vi "参数设置页.vi"() -> ()   [LabVIEW 2016, in "斯坦道总磷总氮.lvlib"]
uses:
  <vilib>/Plasmionique/MB Master/MB_Master/MB_Master.lvclass
  <vilib>/ptbypt/NI_PtbyPt.lvlib
  <vilib>/Plasmionique/MB Master/MB Master.lvlib
panel:
  in  "手动模式":bool caption="手动模式(hd)"
  in  "简易流程周期设置":cluster{"switch button":bool, "设置按钮":bool}
  out "连接状态":bool
  in  "标样核查自动补测":bool caption="通讯连接"
  in  "跨度核查自动补测":bool caption="通讯连接"
  in  "零点核查自动补测":bool caption="通讯连接"
  in  "标样核查标液偏差":dbl caption="标样核查标液偏差："
  in  "跨度核查标液偏差":dbl caption="跨度核查标液偏差："
  in  "零点核查标液偏差":dbl caption="零点核查标液偏差："
  out "低量程上限":dbl caption="低量程上限：" format="%#_g mg/L"
  in  "简易流程路径":path=path "data/流程.xml"
  out "数据刷新时间":string
  in  "通讯连接":bool=TRUE
  out "MB table":enum32{"Serial", "TCP"}(tab)
  in  "请选择串口:":refnum<visa-resource-name>
  in  "协议":u16(ring)=1 caption="协         议:" items=["斯坦道协议"=1, "国标协议"=2]
  in  "波   特   率:":u32(ring)=115200 items=["115200"=115200, "9600"=9600]
  in  "IP":string="127.0.0.1"
  in  "PORT":string="1001"
  in  "通信方式选择":enum16{"串口", "TCP"}(ring)
  in  "盐度自动补偿：":bool
  out "盐度补偿值":dbl caption="盐度补偿值：" format="%#_g ppt"
  in  "刷新":bool
  in  "测量模式":T1(ring)
  in  "参数下拉列表":u16(ring)
  in  "量程下拉列表":enum16{"低量程", "高量程"}(ring)
  in  "测试流程路径":path=path "data/流程.xml"
  in  "标样核查量程模式":T2 caption="标样核查："
  in  "加标回收量程模式":T2 caption="加标回收："
  in  "跨度核查量程模式":T2 caption="跨度核查："
  in  "零点核查量程模式":T2 caption="零点核查："
  in  "水样测试量程模式":T2 caption="水样测试："
  out "稀释度":dbl caption="稀释度："
  out "阈值（高->低）":dbl caption="阈值（高->低）：" format="%#_g mg/L"
  out "阈值（低->高）":dbl caption="阈值（低->高）：" format="%#_g mg/L"
  out "量程下限":dbl caption="量程下限：" format="%#_g mg/L"
  out "高量程上限":dbl caption="高量程上限：" format="%#_g mg/L"
  out "检出限":dbl caption="检出限：" format="%#_g mg/L"
  out "曲线截距":dbl caption="曲线截距：" format="%#.6f"
  out "曲线斜率":dbl caption="曲线斜率：" format="%#.6f"
  out "二次多项式系数":dbl caption="二次多项式系数：" format="%#.6f"
  out "消解时长":dbl caption="消解时长：" format="%#_g min"
  out "消解温度":dbl caption="消解温度：" format="%#_g ℃"
  out "测量精度":u16 caption="测量精度："
  in  "标样核查标液浓度":dbl caption="标样核查标液浓度："
  in  "跨度核查标液浓度":dbl caption="跨度核查标液浓度："
  in  "零点核查标液浓度":dbl caption="零点核查标液浓度："
  in  "跨度值":dbl caption="跨度值："
  # "日质控设置"
  # "关键参数"
  # "连接设置"
  # "mg/L"
  # "mg/L"
  # "mg/L"
  # "mg/L"
  # "±"
  # "%"
  # "%"
  # "流程设置"
  # "简易流程周期设置"
  # "自动测试量程设置"
  # "设置："
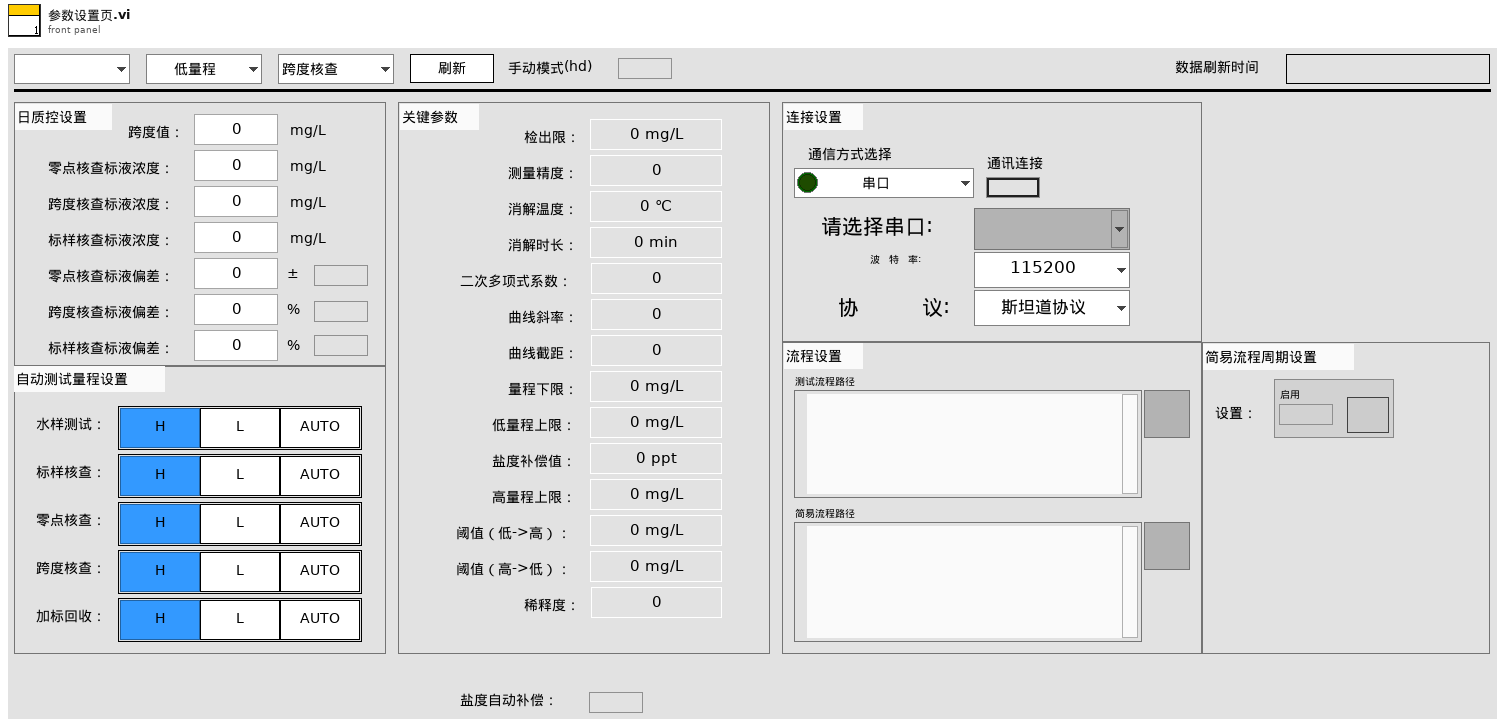
[diagram p1: front panel]
types:
  T1 = enum16{"跨度核查", "水样测量", "零点核查", "标样核查", "加标回收", "平行样测试", "空白校准", "标样校准", "空白测试"}
  T2 = typedef "斯坦道总磷总氮.lvlib/量程模式.ctl" = enum32{"H", "L", "AUTO"}
  T3 = typedef "Cleaning cycle.lvclass/周期项.ctl" = cluster{"时":i32, "分":i32, "频次":string, "id":i32, "参数":string, "simpleflowid":i32, "简易流程名称":string}
  T4 = cluster{"系统时间":timestamp, "工作状态":u16, "测量模式":enum16{"待机", "连续模式", "周期模式", "定点模式", "受控模式", "手动模式"}, "告警代码":u16, "故障代码":u16, "日志代码":u16, "软件版本":u16, "F0":sgl, "F1":sgl, "F2":sgl, "F3":sgl, "T":sgl, "H":sgl, "id":u16, "flowid":u16, "量程":u16, "总磷控温温度1":sgl, "营养盐控温温度2":sgl, "ADC":sgl, "结果值":sgl, "运行时间":u16, "步骤详情":string, "步骤流程":string}
  T5 = typedef "LVStringsAndValuesArrayTypeDef_U16.ctl" = cluster{"String":string, "Value":u16}[]
  T6 = enum8{"Enabled", "Disabled", "Disabled and Grayed Out"}
  T7 = cluster{"测量精度":u16, "检出限":dbl, "上限":dbl, "下限":dbl, "阈值（低->高）":dbl, "阈值（高->低）":dbl, "稀释度":dbl}
  T8 = typedef "操作日志字段定义.ctl" = cluster{"时间":timestamp, "参数":string, "日志信息":string, "流程参数":string}
  T9 = typedef "SingleStepTestV3.lvlib/SingleStepTestV3.lvclass/仪器版本.ctl" = enum16{"V3.1版", "V4版", "V3版", "V4.2版"}
  T10 = typedef "斯坦道总磷总氮.lvlib/V3.1版外设参数.ctl" = cluster{"泵类型":u8, "进样速度":u32, "出样速度":u32, "泵阀量":u8, "阀方向":u8, "光谱仪类型":u8, "光谱采样次数":u8, "氙灯次数":u8, "B":u16, "C":u16, "D":u16, "E":u16, "B_COD":u16, "C_COD":u16, "D_COD":u16, "E_COD":u16, "G":u16, "M":u16, "N":u16, "氨氮注射泵控温下限":sgl, "氨氮注射泵控温上限":sgl, "总氮注射泵控温下限":sgl, "总氮注射泵控温上限":sgl, "消解温度下限":sgl, "消解温度上限":sgl, "加热10s限值":sgl, "KP":sgl, "KI":sgl, "KD":sgl, "高温高压阀开阀温度":sgl, "总氮x公式0":u8, "总氮x公式1":sgl, "总氮x公式2":sgl, "总磷浊度稀释系数":sgl, "总磷浊度补偿权重1":sgl, "总磷浊度补偿权重2":sgl, "盐度系数":sgl, "氨氮补偿系数1":sgl, "氨氮补偿系数2":sgl}
  T11 = typedef "斯坦道总磷总氮.lvlib/V4版外设参数.ctl" = cluster{"泵类型":u8, "注射泵正常速度":u32, "注射泵慢速":u32, "阀型号":u8, "res":u8, "光谱仪类型":u8, "光谱采样次数":u8, "氙灯次数":u8, "B":u16, "C":u16, "D":u16, "E":u16, "B_COD":u16, "C_COD":u16, "D_COD":u16, "E_COD":u16, "G":u16, "M":u16, "N":u16, "降温下限":sgl, "降温上限":sgl, "恒温温度下限":sgl, "恒温温度上限":sgl, "消解温度下限":sgl, "消解温度上限":sgl, "加热10s限值":sgl, "KP":sgl, "KI":sgl, "KD":sgl, "高温高压阀开阀温度":sgl, "总氮x公式0":u8, "总氮x公式1":sgl, "总氮x公式2":sgl, "总磷浊度稀释系数":sgl, "总磷浊度补偿权重1":sgl, "总磷浊度补偿权重2":sgl, "盐度系数":sgl, "氨氮补偿系数1":sgl, "氨氮补偿系数2":sgl, "缺试剂传感器阈值":u16}
  T12 = typedef "斯坦道总磷总氮.lvlib/V4.2版外设参数.ctl" = cluster{"工作模式":u16, "泵类型":u16, "阀型号":u16, "注射泵进样速度":u16, "注射泵出样速度":u16, "注射泵滴定速度":u16, "res":u16, "注射泵慢速":u16, "光谱仪类型":u16, "光谱采样次数":u16, "氙灯次数":u16, "B":u16, "C":u16, "D":u16, "E":u16, "B_COD":u16, "C_COD":u16, "D_COD":u16, "E_COD":u16, "G":u16, "M":u16, "N":u16, "温度校准参数":sgl, "降温温度":sgl, "恒温温度":sgl, "消解温度":sgl, "高温高压阀开阀温度":sgl, "加热超时时间":sgl, "KP":sgl, "KI":sgl, "KD":sgl, "消解PID积分上限":sgl, "恒温PID积分上限":sgl, "PID积分下限":sgl, "缺试剂传感器阈值":u16, "滴定延时":u16, "滴定斜率阈值":sgl, "总氮x公式0":u16, "总氮x公式1":sgl, "总氮x公式2":sgl, "总磷浊度稀释系数":sgl, "总磷浊度补偿权重1":sgl, "总磷浊度补偿权重2":sgl, "盐度系数":sgl, "氨氮补偿系数1":sgl, "氨氮补偿系数2":sgl}
  T13 = typedef "斯坦道总磷总氮.lvlib/V3版外设参数.ctl" = cluster{"泵类型":u8, "进样速度":u32, "出样速度":u32, "泵阀量":u8, "光谱仪类型":u8, "光谱采样次数":u8, "氙灯次数":u8, "B":u16, "C":u16, "D":u16, "E":u16, "B_COD":u16, "C_COD":u16, "D_COD":u16, "E_COD":u16, "G":u16, "M":u16, "N":u16, "氨氮注射泵控温下限":sgl, "氨氮注射泵控温上限":sgl, "总氮注射泵控温下限":sgl, "总氮注射泵控温上限":sgl, "消解温度下限":sgl, "消解温度上限":sgl, "加热10s限值":sgl, "高温高压阀开阀温度":sgl, "总氮x公式0":u8, "总氮x公式1":sgl, "总氮x公式2":sgl, "总磷浊度稀释系数":sgl, "总磷浊度补偿权重1":sgl, "总磷浊度补偿权重2":sgl, "盐度系数":sgl, "氨氮补偿系数1":sgl, "氨氮补偿系数2":sgl}
  T14 = cluster{"水样测试量程模式":T2, "零点核查量程模式":T2, "跨度核查量程模式":T2, "加标回收量程模式":T2, "标样核查量程模式":T2}
  T15 = cluster{"总磷":dbl, "总氮":dbl, "氨氮":dbl, "磷酸盐":dbl, "硝氮":dbl, "亚硝氮":dbl, "硅酸盐":dbl, "硫化物":dbl, "COD":dbl, "氟化物":dbl, "CODMn":dbl}
  T16 = cluster{"总磷跨度值":dbl, "总磷零点标准液浓度":dbl, "总磷跨度标准液浓度":dbl, "总磷标准液标准浓度":dbl, "总氮跨度值":dbl, "总氮零点标准液浓度":dbl, "总氮跨度标准液浓度":dbl, "总氮标准液标准浓度":dbl, "COD跨度值":dbl, "COD零点标准液浓度":dbl, "COD跨度标准液浓度":dbl, "COD标准液标准浓度":dbl, "氨氮跨度值":dbl, "氨氮零点标准液浓度":dbl, "氨氮跨度标准液浓度":dbl, "氨氮标准液标准浓度":dbl, "磷酸盐跨度值":dbl, "磷酸盐零点标准液浓度":dbl, "磷酸盐跨度标准液浓度":dbl, "磷酸盐标准液标准浓度":dbl, "硝氮跨度值":dbl, "硝氮零点标准液浓度":dbl, "硝氮跨度标准液浓度":dbl, "硝氮标准液标准浓度":dbl, "亚硝氮跨度值":dbl, "亚硝氮零点标准液浓度":dbl, "亚硝氮跨度标准液浓度":dbl, "亚硝氮标准液标准浓度":dbl, "硫化物跨度值":dbl, "硫化物零点标准液浓度":dbl, "硫化物跨度标准液浓度":dbl, "硫化物标准液标准浓度":dbl, "硅酸盐跨度值":dbl, "硅酸盐零点标准液浓度":dbl, "硅酸盐跨度标准液浓度":dbl, "硅酸盐标准液标准浓度":dbl, "总磷零点标准液偏差":dbl, "总磷跨度标准液偏差":dbl, "总磷标准液标准偏差":dbl, "总氮零点标准液偏差":dbl, "总氮跨度标准液偏差":dbl, "总氮标准液标准偏差":dbl, "COD零点标准液偏差":dbl, "COD跨度标准液偏差":dbl, "COD标准液标准偏差":dbl, "氨氮零点标准液偏差":dbl, "氨氮跨度标准液偏差":dbl, "氨氮标准液标准偏差":dbl, "磷酸盐零点标准液偏差":dbl, "磷酸盐跨度标准液偏差":dbl, "磷酸盐标准液标准偏差":dbl, "硝氮零点标准液偏差":dbl, "硝氮跨度标准液偏差":dbl, "硝氮标准液标准偏差":dbl, "亚硝氮零点标准液偏差":dbl, "亚硝氮跨度标准液偏差":dbl, "亚硝氮标准液标准偏差":dbl, "硫化物零点标准液偏差":dbl, "硫化物跨度标准液偏差":dbl, "硫化物标准液标准偏差":dbl, "硅酸盐零点标准液偏差":dbl, "硅酸盐跨度标准液偏差":dbl, "硅酸盐标准液标准偏差":dbl, "氟化物跨度值":dbl, "氟化物零点标准液浓度":dbl, "氟化物跨度标准液浓度":dbl, "氟化物标准液标准浓度":dbl, "氟化物零点标准液偏差":dbl, "氟化物跨度标准液偏差":dbl, "氟化物标准液标准偏差":dbl, "CODMn跨度值":dbl, "CODMn零点标准液浓度":dbl, "CODMn跨度标准液浓度":dbl, "CODMn标准液标准浓度":dbl, "CODMn零点标准液偏差":dbl, "CODMn跨度标准液偏差":dbl, "CODMn标准液标准偏差":dbl}
  T17 = cluster{"测量精度":u16, "消解温度":u16, "消解时长":u16, "量程下限":sgl, "量程上限":sgl, "曲线斜率K":sgl, "曲线斜率B":sgl, "标定日期":timestamp, "标液1浓度":sgl, "标液1测量过程值":sgl, "标液2浓度":sgl, "标液2测量过程值":sgl, "标液3浓度":sgl, "标液3测量过程值":sgl, "标液4浓度":sgl, "标液4测量过程值":sgl, "标液5浓度":sgl, "标液5测量过程值":sgl, "线性相关系数":sgl, "试剂余量":u32, "测量滴定值或吸光度":sgl, "空白校准时间":timestamp, "标样校准时间":timestamp, "检出限值":sgl, "校准系数":sgl, "设备系列号":string}
  T18 = cluster{"水样测试量程模式":enum16{"H", "L", "AUTO"}, "空白核查量程模式":enum16{"H", "L", "AUTO"}, "跨度核查量程模式":enum16{"H", "L", "AUTO"}, "加标回收量程模式":enum16{"H", "L", "AUTO"}, "标样核查量程模式":enum16{"H", "L", "AUTO"}}
  T19 = cluster{"水样测试量程模式":u16, "空白核查量程模式":u16, "跨度核查量程模式":u16, "加标回收量程模式":u16, "标样核查量程模式":u16}
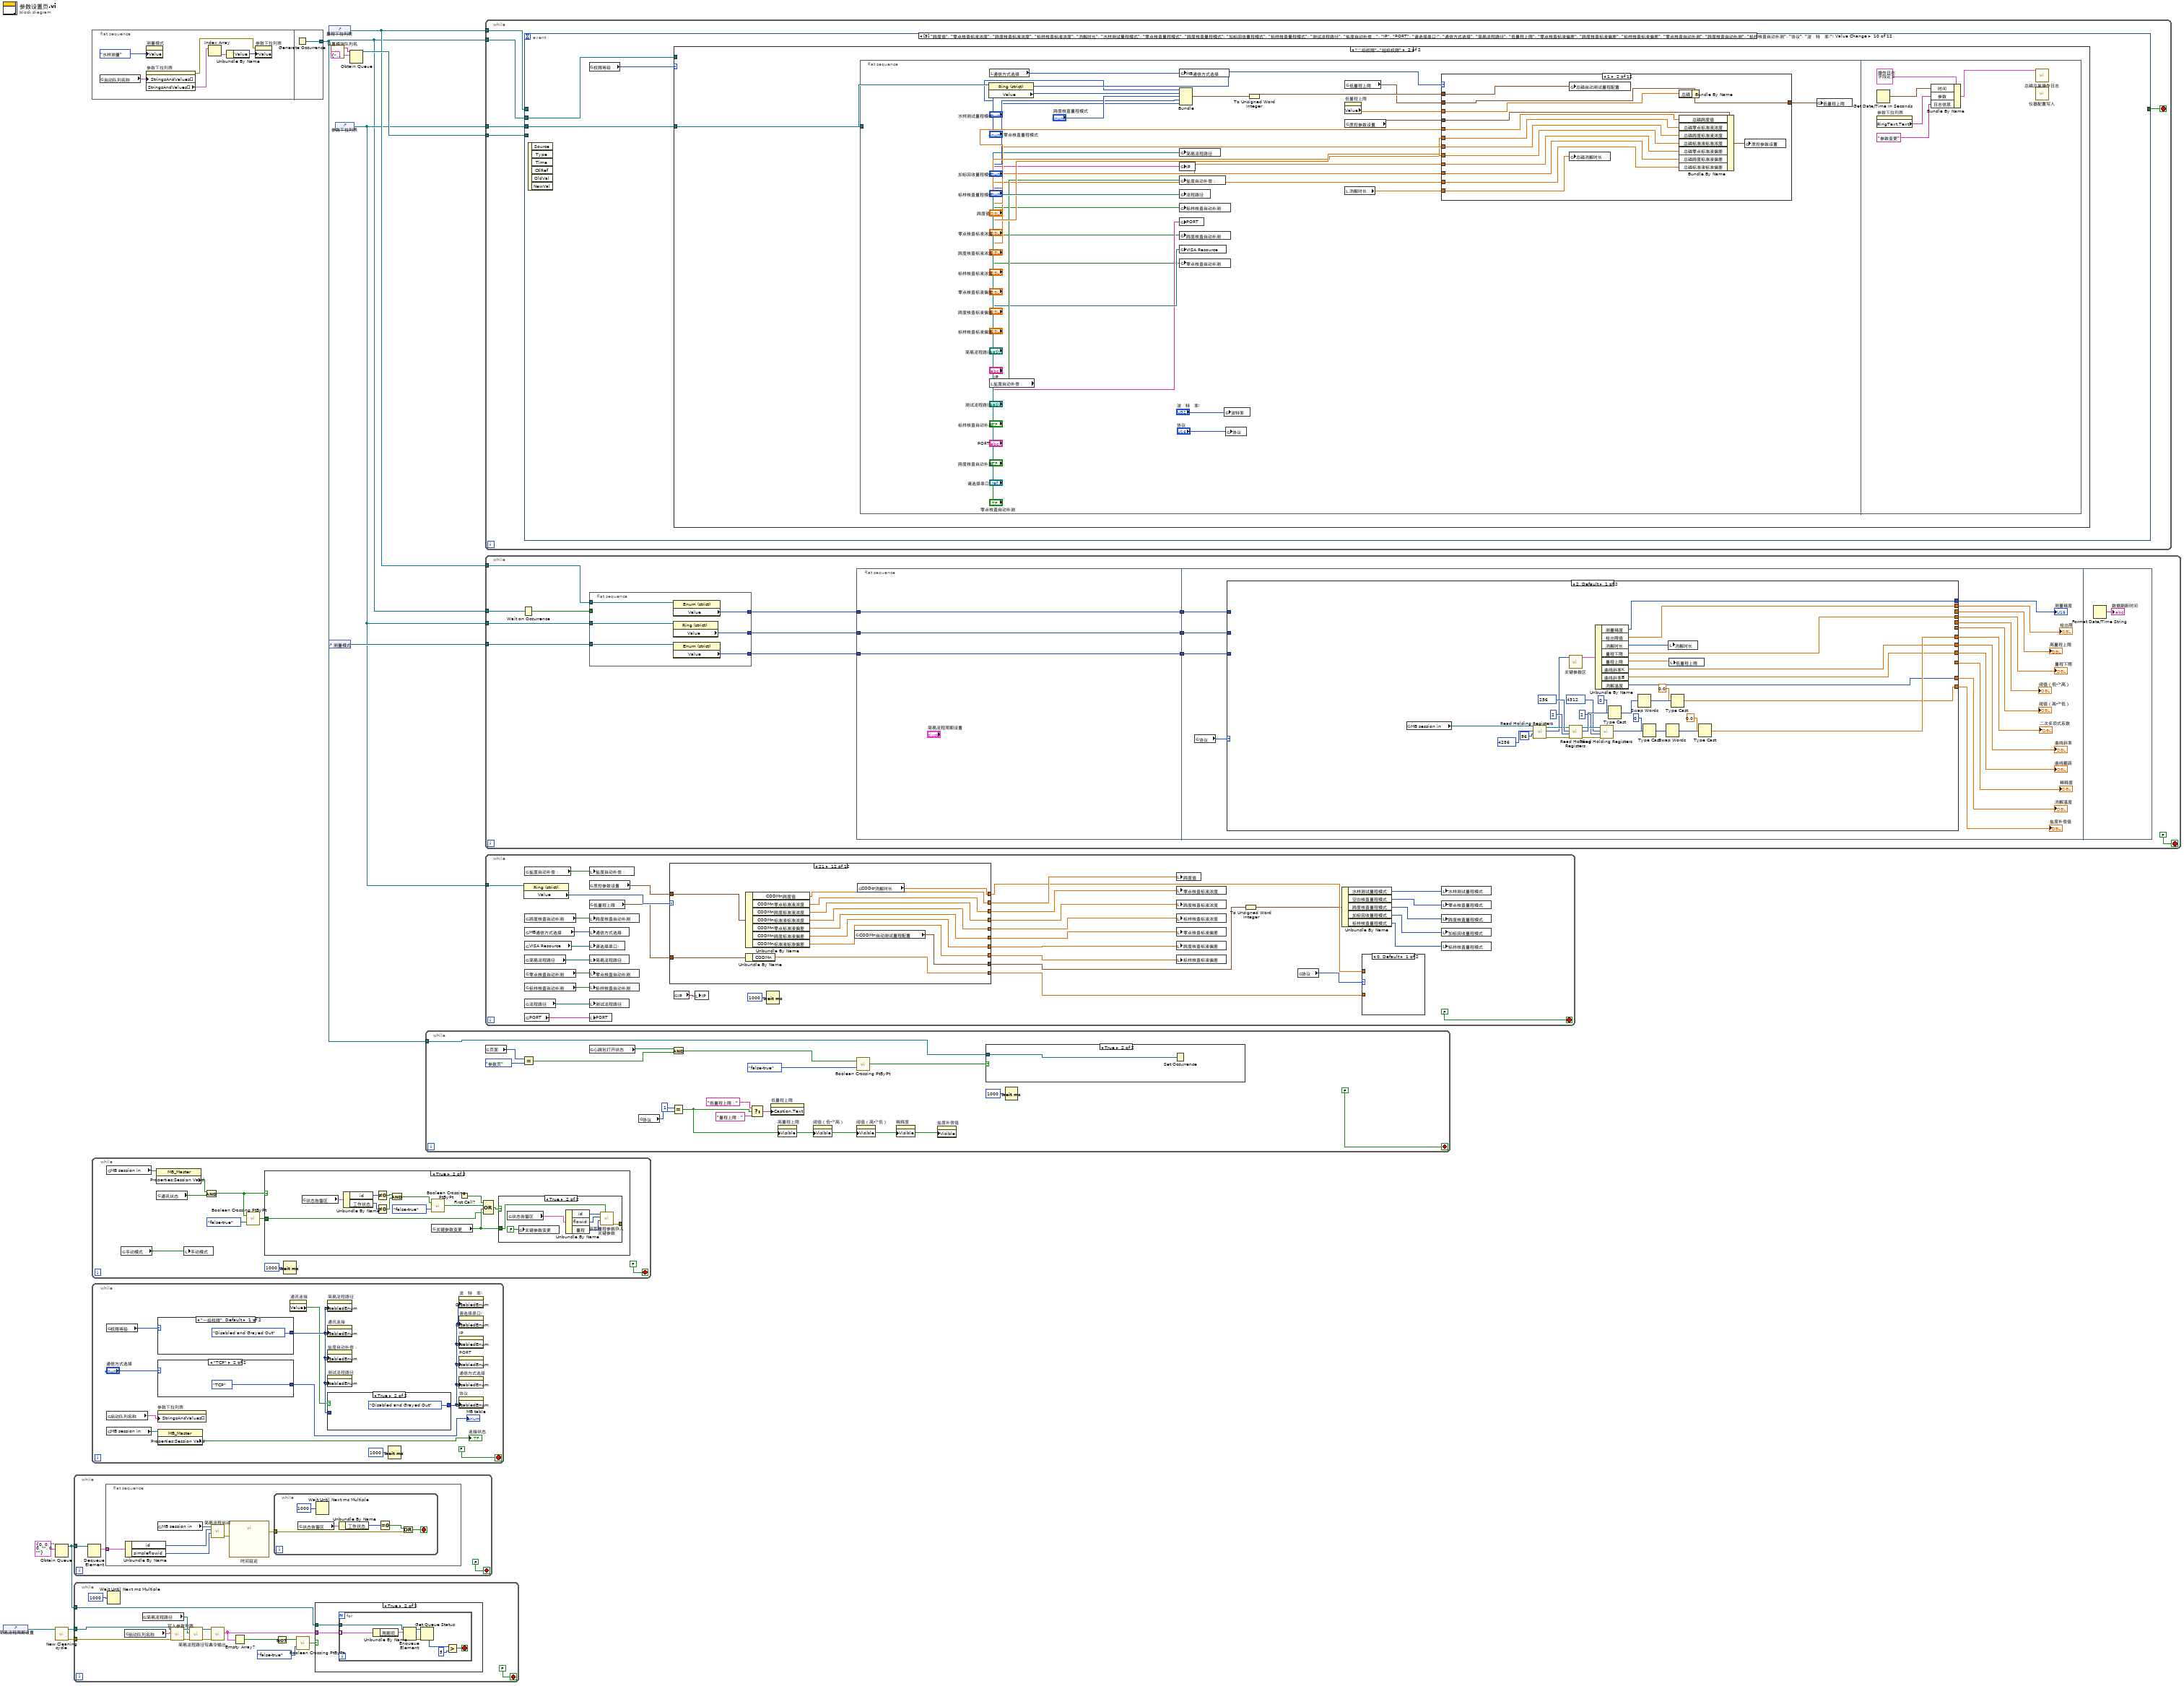
[diagram p0: block diagram]
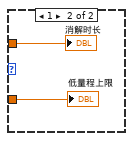
[diagram p6: hidden frame]
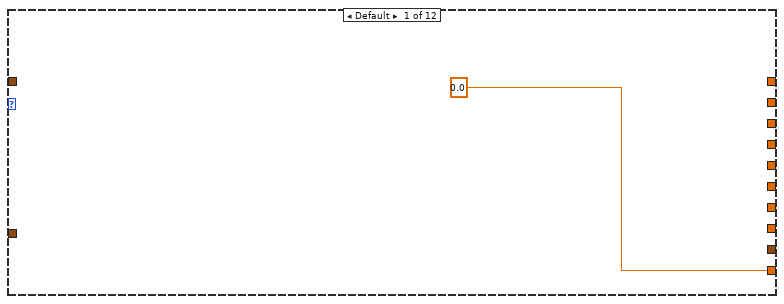
[diagram p7: hidden frame]
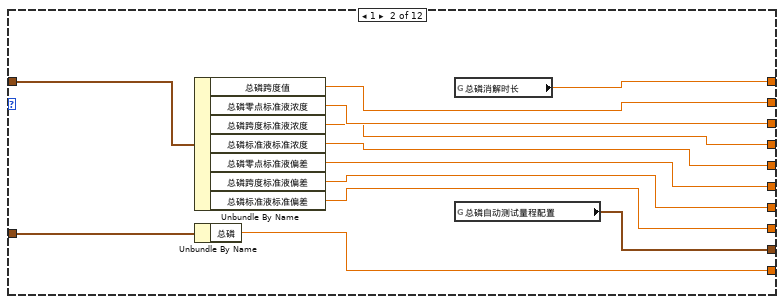
[diagram p8: hidden frame]
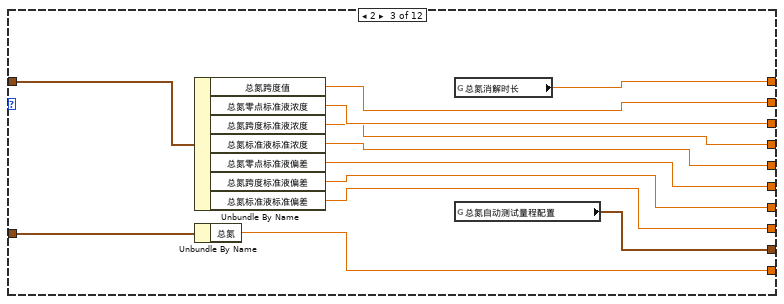
[diagram p9: hidden frame]
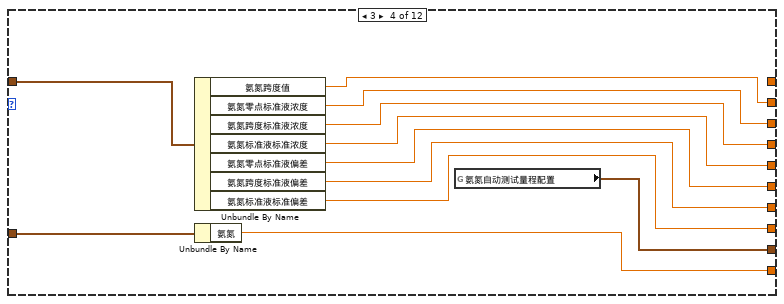
[diagram p10: hidden frame]
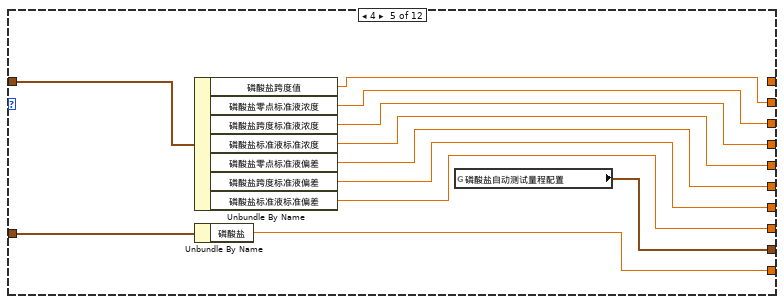
[diagram p11: hidden frame]
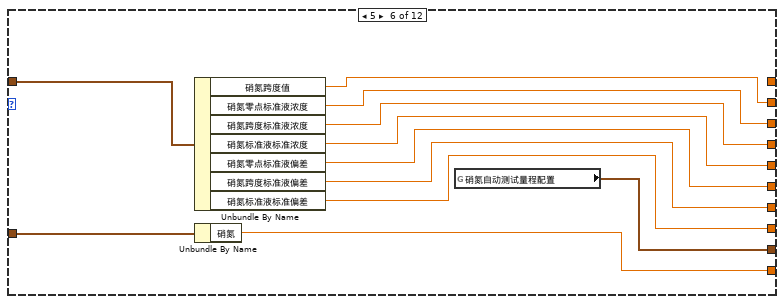
[diagram p12: hidden frame]
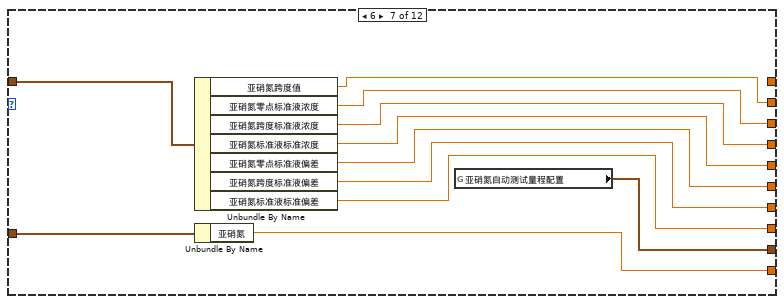
[diagram p13: hidden frame]
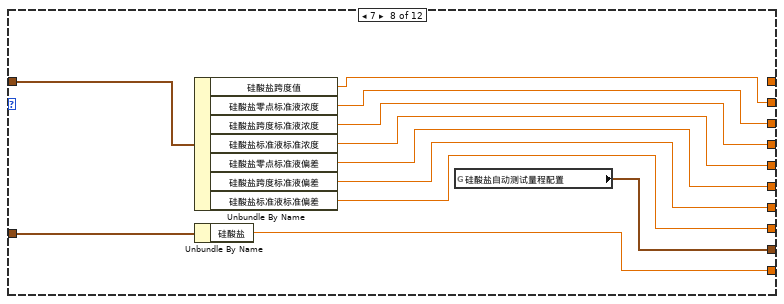
[diagram p14: hidden frame]
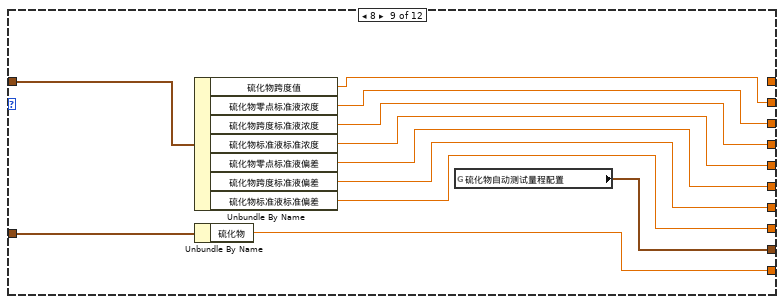
[diagram p15: hidden frame]
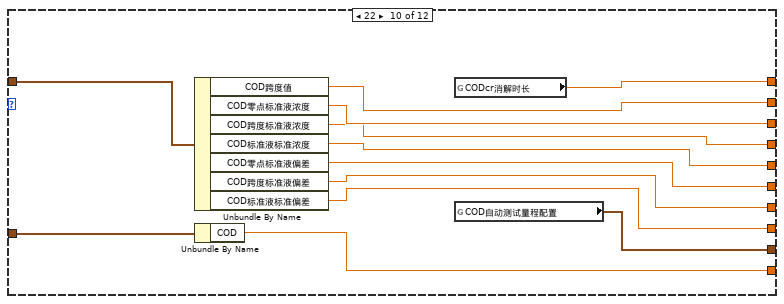
[diagram p16: hidden frame]
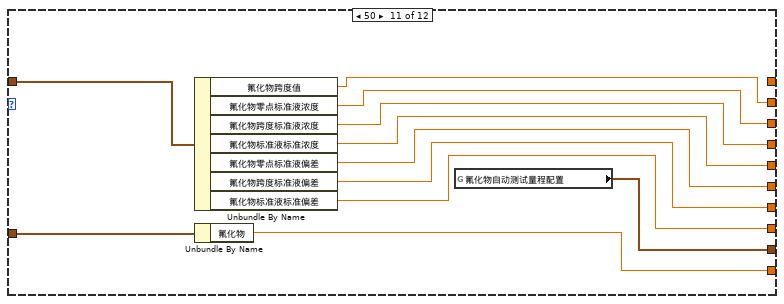
[diagram p17: hidden frame]
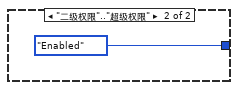
[diagram p18: hidden frame]
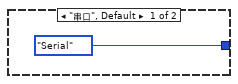
[diagram p19: hidden frame]
diagram:
  n1 = control-ref of="简易流程周期设置"() -> (w3:refnum<vi>)
  n2 = Obtain Queue(element data type=T3 {"时"=0, "分"=0, "频次"="", "id"=0, "参数"="", "simpleflowid"=0, "简易流程名称"=""} ("周期项")) -> (queue out=w1:refnum<queue>)  [unwired: 4 in, 2 out]
  n3 = call "New Cleaning cycle.vi"("Reference"=w3) -> ("error out"=w4:errorcluster, "Cleaningcycle out"=w5:refnum<class "Cleaning cycle.lvclass">)  [unwired: 9 in]
  n4 = while {
    tunnel: w1 -> [w15]
    stop <- FALSE stop-if-true
    n5 = Dequeue Element(queue=w15) -> (element=w14:T3)  [unwired: 2 in, 3 out]
    n6 = flat-sequence {
      tunnel: w14 -> [w20]
      frame #0 {
        n7 = Unbundle By Name(w20) -> ("id"=w18:i32, "simpleflowid"=w19:i32)
        n8 = global read "VAR总磷总氮全局变量.vi" "MB session in"() -> (w21:refnum<class "MB_Master.lvclass">)
        n9 = call "简易流程启动.vi"("简易流程"=w19, "参数Id"=w18, "MB session in"=w21) -> ("error out"=w17:errorcluster)  [unwired: 7 in, 1 out]
        n10 = call "时间延迟"("error in (no error)"=w17) -> ("error out"=w16:errorcluster)  [unwired: 10 in]
        n11 = while {
          tunnel: w16 -> [w23]
          stop <- w22 stop-if-true
          n12 = global read "VAR总磷总氮全局变量.vi" "状态告警区"() -> (w26:T4)
          n13 = Wait Until Next ms Multiple(millisecond multiple=u32 1000 ("毫秒倍数")) -> ()  [unwired: 1 out]
          n14 = Unbundle By Name(w26) -> ("工作状态"=w25:u16)
          n15 = Equal To 0?(x=w25) -> (x = 0?=w24:bool)
          n16 = Or(x=w24, y=w23) -> (x .or. y?=w22:bool)
        }
      }
    }
  }
  n17 = while {
    tunnel: w5 -> [w43]
    tunnel: w4 -> [w42]
    tunnel: w1 -> [w29]
    stop <- FALSE stop-if-true
    n18 = Wait Until Next ms Multiple(millisecond multiple=u32 1000 ("毫秒倍数")) -> ()  [unwired: 1 out]
    n19 = global read "model config var.vi" "启动队列名称"() -> (w39:cluster{"String":string, "Value":u16}[])
    n20 = global read "总磷总氮断电保存全局变量.vi" "简易流程路径"() -> (w38:path)
    n21 = call "写入参数列表.vi"("error in (no error)"=w42, "参数列表"=w39, "Cleaningcycle 输入"=w43) -> ("error out"=w41:errorcluster, "Cleaningcycle 输出"=w40:refnum<class "Cleaning cycle.lvclass">)  [unwired: 7 in]
    n22 = call "简易流程路径写入.vi"("error in (no error)"=w41, "简易流程路径"=w38, "Cleaningcycle 输入"=w40) -> ("error out"=w36:errorcluster, "Cleaningcycle 输出"=w37:refnum<class "Cleaning cycle.lvclass">)  [unwired: 7 in]
    n23 = call "命令输出.vi"("error in (no error)"=w36, "Cleaningcycle 输入"=w37) -> ("命令"=w31:cluster{"触发":bool, "周期项":T3}[])  [unwired: 7 in, 2 out]
    n24 = Empty Array?(array=w31) -> (empty?=w35:bool)
    n25 = Not(x=w35) -> (.not. x?=w34:bool)
    n26 = call <vilib>:"Boolean Crossing PtByPt.vi"("direction"=enum16{"either", "false-true", "true-false"}."false-true", "input"=w34) -> ("crossing"=w32:bool)  [unwired: 1 in]
    n27 = case shown="True" w32 {
      tunnel: w31 -> [_ w45]
      tunnel: w29 -> [_ w44]
      frame False {
      }
      frame True {
        n28 = for {
          tunnel: w45 -> [w53] mode=indexing
          tunnel: w44 -> [w51]
          stop <- w46 stop-if-true
          n29 = Unbundle By Name(w53) -> ("周期项"=w52:T3)
          n30 = Enqueue Element(queue=w51, element=w52) -> (queue out=w50:refnum<queue>, error out=w49:errorcluster)  [unwired: 2 in, 1 out]
          n31 = Get Queue Status(queue=w50, error in (no error)=w49) -> (# elements in queue=w48:i32)  [unwired: 1 in, 7 out]
          n32 = Greater?(x=w48, y=5) -> (0:w46:bool)
        }
      }
    }
  }
  n33 = flat-sequence {
    tunnel: [w60] -> w6
    frame #0 {
      n34 = global read "model config var.vi" "启动队列名称"() -> (w55:cluster{"String":string, "Value":u16}[])
      n35 = property on="测量模式" class="Enum (strict)"("Value"=T1."水样测量" ("测量模式")) -> ()  [unwired: 2 in, 2 out]
      n36 = property on="参数下拉列表" class="Ring (strict)"("StringsAndValues[]"=w55) -> (error out=w58:errorcluster, "StringsAndValues[]"=w56:T5)  [unwired: 2 in, 1 out]
      n37 = Index Array(array=w56) -> (element=w57:cluster{"String":string, "Value":u16})  [unwired: 1 in]
      n38 = Unbundle By Name(w57) -> ("Value"=w59:u16)
      n39 = property on="参数下拉列表" class="Ring (strict)"(error in=w58, "Value"=w59) -> ()  [unwired: 1 in, 2 out]
    }
    frame #1 {
      n40 = Generate Occurrence() -> (w60:refnum<k4>)
    }
  }
  n41 = while {
    stop <- FALSE stop-if-true
    n42 = global read "VAR总磷总氮全局变量.vi" "MB session in"() -> (w66:refnum<class "MB_Master.lvclass">)
    n43 = global read "VAR总磷总氮全局变量.vi" "手动模式"() -> (w61:bool)
    n44 = property class="MB_Master"(reference=w66) -> ("Properties:Session Valid"=w65:bool)  [unwired: 1 in, 2 out]
    n45 = global read "VAR总磷总氮全局变量.vi" "通讯状态"() -> (w68:bool)
    n46 = local write "手动模式"(w61) -> ()
    n47 = And(x=w65, y=w68) -> (x .and. y?=w63:bool)
    n48 = call <vilib>:"Boolean Crossing PtByPt.vi"("direction"=enum16{"either", "false-true", "true-false"}."false-true", "input"=w63) -> ("crossing"=w62:bool)  [unwired: 1 in]
    n49 = case shown="True" w63 {
      tunnel: w62 -> [_ w71]
      frame False {
      }
      frame True {
        n50 = global read "VAR总磷总氮全局变量.vi" "状态告警区"() -> (w81:T4)
        n51 = Unbundle By Name(w81) -> ("id"=w75:u16, "工作状态"=w80:u16)
        n52 = Not Equal To 0?(x=w75) -> (x != 0?=w76:bool)
        n53 = Not Equal To 0?(x=w80) -> (x != 0?=w77:bool)
        n54 = And(x=w76, y=w77) -> (x .and. y?=w78:bool)
        n55 = call <vilib>:"Boolean Crossing PtByPt.vi"("direction"=enum16{"either", "false-true", "true-false"}."false-true", "input"=w78) -> ("crossing"=w74:bool)  [unwired: 1 in]
        n56 = global read "VAR总磷总氮全局变量.vi" "关键参数变更"() -> (w72:bool)
        n57 = First Call?() -> (First Call?: T/F=w70:bool)
        n58 = Compound Arithmetic op=OR ("复合运算")(w70, w74, w72, w71) -> (w73:bool)
        n59 = case shown="True" w73 {
          tunnel: [_ w88] -> _
          tunnel: w72 -> [_ w83]
          frame False {
          }
          frame True {
            n60 = global read "VAR总磷总氮全局变量.vi" "状态告警区"() -> (w87:T4)
            n61 = global write "VAR总磷总氮全局变量.vi" "关键参数变更"(FALSE ("关键参数变更")) -> ()
            n62 = Unbundle By Name(w87) -> ("id"=w86:u16, "flowid"=w85:u16, "量程"=w84:u16)
            n63 = call "获取量程参数存入关键参数.vi"("关键参数变更"=w83, "量程"=w84, "flowid"=w85, "id"=w86) -> ("error out"=w88:errorcluster)  [unwired: 7 in]
          }
        }
      }
    }
    n64 = Wait (ms)(milliseconds to wait=u32 1000 ("等待时间（毫秒）")) -> ()  [unwired: 1 out]
  }
  n65 = while {
    stop <- FALSE stop-if-true
    n66 = global read "VAR总磷总氮全局变量.vi" "权限等级"() -> (w94:enum16{"一级权限", "二级权限", "三级权限", "超级权限"})
    n67 = global read "model config var.vi" "启动队列名称"() -> (w92:cluster{"String":string, "Value":u16}[])
    n68 = global read "VAR总磷总氮全局变量.vi" "MB session in"() -> (w98:refnum<class "MB_Master.lvclass">)
    n69 = case shown="\"一级权限\", Default" w94 {
      tunnel: [T6."Disabled and Grayed Out" ("禁用") T6."Enabled" ("禁用")] -> w93
      frame "一级权限", Default {
      }
      frame "二级权限".."超级权限" {
      }
    }
    n70 = case shown="\"TCP\"" "通信方式选择" {
      tunnel: [enum32{"Serial", "TCP"}."Serial" ("MB table") enum32{"Serial", "TCP"}."TCP" ("MB table")] -> w96
      frame "串口", Default {
      }
      frame "TCP" {
      }
    }
    "MB table" <- w96
    n71 = property on="参数下拉列表" class="Ring (strict)"("StringsAndValues[]"=w92) -> ()  [unwired: 2 in, 2 out]
    n72 = property class="MB_Master"(reference=w98) -> ("Properties:Session Valid"=→"连接状态":bool)  [unwired: 1 in, 2 out]
    n73 = property on="通讯连接" class="Bool (strict)"() -> ("Value"=w90:bool)  [unwired: 2 in, 2 out]
    n74 = property on="简易流程路径" class="Path"("DisabledEnum"=w93) -> ()  [unwired: 2 in, 2 out]
    n75 = property on="通讯连接" class="Bool (strict)"("DisabledEnum"=w93) -> ()  [unwired: 2 in, 2 out]
    n76 = property on="盐度自动补偿：" class="Bool (strict)"("DisabledEnum"=w93) -> ()  [unwired: 2 in, 2 out]
    n77 = property on="测试流程路径" class="Path"("DisabledEnum"=w93) -> ()  [unwired: 2 in, 2 out]
    n78 = case shown="True" w90 {
      tunnel: [w104 T6."Disabled and Grayed Out" ("禁用")] -> w89
      tunnel: w93 -> [w104 _]
      frame False {
      }
      frame True {
      }
    }
    n79 = Wait (ms)(milliseconds to wait=u32 1000 ("等待时间（毫秒）")) -> ()  [unwired: 1 out]
    n80 = property on="波   特   率:" class="Ring (strict)"("DisabledEnum"=w89) -> ()  [unwired: 2 in, 2 out]
    n81 = property on="请选择串口:" class="VISAName"("DisabledEnum"=w89) -> ()  [unwired: 2 in, 2 out]
    n82 = property on="IP" class="Str"("DisabledEnum"=w89) -> ()  [unwired: 2 in, 2 out]
    n83 = property on="PORT" class="Str"("DisabledEnum"=w89) -> ()  [unwired: 2 in, 2 out]
    n84 = property on="通信方式选择" class="Enum (strict)"("DisabledEnum"=w89) -> ()  [unwired: 2 in, 2 out]
    n85 = property on="协议" class="Ring (strict)"("DisabledEnum"=w89) -> ()  [unwired: 2 in, 2 out]
  }
  n86 = control-ref of="量程下拉列表"() -> (w8:refnum<vi>)
  n87 = control-ref of="测量模式"() -> (w9:refnum<vi>)
  n88 = call "设置模块队列名.vi"() -> ("Msg"=w11:string)  [unwired: 5 in]
  n89 = control-ref of="参数下拉列表"() -> (w7:refnum<vi>)
  n90 = Obtain Queue(name (unnamed)=w11, element data type=cluster{"命令":string, "data":variant} {"命令"="", "data"=variant}) -> (queue out=w10:refnum<queue>)  [unwired: 3 in, 2 out]
  n91 = while {
    tunnel: w6 -> [w118]
    stop <- FALSE stop-if-true
    n92 = global read "VAR总磷总氮全局变量.vi" "页面"() -> (w120:enum16{"主页", "参数页", "校准页"})
    n93 = Equal?(x=w120, y=enum16{"主页", "参数页", "校准页"}."参数页" ("页面")) -> (x = y?=w119:bool)
    n94 = global read "VAR总磷总氮全局变量.vi" "心跳包打开状态"() -> (w114:bool)
    n95 = global read "总磷总氮断电保存全局变量.vi" "协议"() -> (w107:u16)
    n96 = And(x=w114, y=w119) -> (x .and. y?=w115:bool)
    n97 = Equal?(x=u16 1, y=w107) -> (x = y?=w108:bool)
    n98 = Select(t="低量程上限：" ("标题.文本"), s=w108, f="量程上限：" ("标题.文本")) -> (s? t:f=w109:string)
    n99 = property on="低量程上限" class="DigNum (strict)"("Caption.Text"=w109) -> ()  [unwired: 2 in, 2 out]
    n100 = property on="高量程上限" class="DigNum (strict)"("Visible"=w108) -> ()  [unwired: 2 in, 2 out]
    n101 = property on="阈值（低->高）" class="DigNum (strict)"("Visible"=w108) -> ()  [unwired: 2 in, 2 out]
    n102 = property on="阈值（高->低）" class="DigNum (strict)"("Visible"=w108) -> ()  [unwired: 2 in, 2 out]
    n103 = call <vilib>:"Boolean Crossing PtByPt.vi"("direction"=enum16{"either", "false-true", "true-false"}."false-true", "input"=w115) -> ("crossing"=w113:bool)  [unwired: 1 in]
    n104 = property on="稀释度" class="DigNum (strict)"("Visible"=w108) -> ()  [unwired: 2 in, 2 out]
    n105 = property on="盐度补偿值" class="DigNum (strict)"("Visible"=w108) -> ()  [unwired: 2 in, 2 out]
    n106 = case shown="True" w113 {
      tunnel: w118 -> [_ w122]
      frame False {
      }
      frame True {
        n107 = Set Occurrence(w122) -> ()
      }
    }
    n108 = Wait (ms)(milliseconds to wait=u32 1000 ("等待时间（毫秒）")) -> ()  [unwired: 1 out]
  }
  n109 = while {
    tunnel: w6 -> [w126]
    tunnel: w7 -> [w125]
    tunnel: w10 -> [w124]
    tunnel: w8 -> [w123]
    stop <- w127 stop-if-true
    n110 = event shown="[9] \"跨度值\", \"零点核查标液浓度\", \"跨度核查标液浓度\", \"标样核查标液浓度\", \"消解时长\", \"水样测试量程模式\", \"零点核查量程模式\", \"跨度核查量程模式\", \"加标回收量程模式\", \"标样核查量程模式\", \"测试流程路径\", \"盐度自动补偿：\", \"IP\", \"PORT\", \"请选择串口:\", \"通信方式选择\", \"简易流程路径\", \"低量程上限\", \"零点核查标液偏差\", \"跨度核查标液偏差\", \"标样核查标液偏差\", \"零点核查自动补测\", \"跨度核查自动补测\", \"标样核查自动补测\", \"协议\", \"波   特   率:\": Value Change" {
      selector: _ -> [_ _ _ _ _ _ _ _ _ _ _ _]
      dyn-events: _ -> [_ _ _ _ _ _ _ _ _ _ _ _]
      timeout: _ -> [_ _ _ _ _ _ _ _ _ _ _ _]
      tunnel: [_ TRUE _ _ _ _ _ _ _ _ _ _] -> w127
      tunnel: w126 -> [_ _ w129 _ _ _ _ _ _ w208 _ _]
      tunnel: w125 -> [_ _ _ _ w148 _ _ _ _ w210 _ _]
      tunnel: w124 -> [_ _ _ _ _ _ _ _ _ _ w400 _]
      tunnel: w123 -> [_ _ _ _ _ _ _ _ _ _ _ _]
      event Timeout {
        n111 = event-data() -> ()  [unwired: 1 in, 3 out]
      }
      event Panel Close {
        n112 = event-data() -> ()  [unwired: 1 in, 4 out]
      }
      event "参数下拉列表", "量程下拉列表", "测量模式", "刷新": Value Change {
        n113 = event-data() -> ()  [unwired: 1 in, 6 out]
        n114 = Set Occurrence(w129) -> ()
      }
      event "跨度值", "零点核查标液浓度", "跨度核查标液浓度", "标样核查标液浓度", "消解温度", "消解时长", "检出限", "高量程上限", "量程下限", "阈值（低->高）", "阈值（高->低）", "稀释度", "低量程上限", "零点核查标液偏差", "跨度核查标液偏差", "标样核查标液偏差": Mouse Down {
        n115 = event-data() -> ("CtlRef"=w131:refnum<vi>)  [unwired: 1 in, 5 out]
        n116 = global read "VAR总磷总氮全局变量.vi" "权限等级"() -> (w130:enum16{"一级权限", "二级权限", "三级权限", "超级权限"})
        n117 = case shown="\"二级权限\"..\"超级权限\"" w130 {
          tunnel: w131 -> [_ w135]
          frame "一级权限", Default {
          }
          frame "二级权限".."超级权限" {
            n118 = property class="DigNum (strict)"(reference=w135) -> (reference out=w133:refnum<vi>, "Value"=w134:dbl)  [unwired: 1 in, 1 out]
            n119 = call "数字键盘.vi"("OldNumber"=w134) -> ("NewNumber"=w132:dbl)
            n120 = property class="DigNum (strict)"(reference=w133, "Val(Sgnl)"=w132) -> ()  [unwired: 1 in, 2 out]
          }
        }
      }
      event "测量精度", "检出限", "高量程上限", "量程下限", "阈值（低->高）", "阈值（高->低）", "稀释度": Value Change {
        n121 = event-data() -> ()  [unwired: 1 in, 6 out]
        n122 = local read "测量精度"() -> (w138:u16)
        n123 = local read "检出限"() -> (w142:dbl)
        n124 = local read "高量程上限"() -> (w144:dbl)
        n125 = local read "量程下限"() -> (w143:dbl)
        n126 = local read "阈值（低->高）"() -> (w141:dbl)
        n127 = local read "阈值（高->低）"() -> (w140:dbl)
        n128 = local read "稀释度"() -> (w139:dbl)
        n129 = property class="Ring (strict)"(reference=w148) -> ("Value"=w147:u16)  [unwired: 1 in, 2 out]
        n130 = Bundle By Name(cluster=T7 {"测量精度"=0, "检出限"=0.0, "上限"=0.0, "下限"=0.0, "阈值（低->高）"=0.0, "阈值（高->低）"=0.0, "稀释度"=0.0} ("量程参数写入"), "测量精度"=w138, "检出限"=w142, "上限"=w144, "下限"=w143, "阈值（低->高）"=w141, "阈值（高->低）"=w140, "稀释度"=w139) -> (w145:T7)
        n131 = call "量程参数写入.vi"("量程参数写入"=w145, "测量参数"=w147) -> ("error out"=w136:errorcluster)  [unwired: 8 in]
        n132 = case shown="No Error" w136 {
          tunnel: ["写入成功" "写入失败"] -> w137
          frame No Error {
            n133 = Get Date/Time In Seconds() -> (seconds since 1Jan1904=w151:timestamp)
            n134 = property on="参数下拉列表" class="Ring (strict)"() -> ("RingText.Text"=w149:string)  [unwired: 2 in, 2 out]
            n135 = Bundle By Name(cluster=T8 {"时间"=timestamp(0 s since 1904-01-01), "参数"="", "日志信息"="", "流程参数"=""} ("data in"), "时间"=w151, "参数"=w149, "日志信息"="关键参数变更") -> (w152:T8)
            n136 = call "总磷总氮操作日志.vi"("data in"=w152) -> ()  [unwired: 10 in, 1 out]
            n137 = global write "VAR总磷总氮全局变量.vi" "关键参数变更"(TRUE ("关键参数变更")) -> ()
          }
          frame Error {
          }
        }
        n138 = One Button Dialog(message=w137) -> ()  [unwired: 1 in, 1 out]
      }
      event "消解温度": Value Change {
        n139 = event-data() -> ("NewVal"=w158:dbl)  [unwired: 1 in, 5 out]
        n140 = global read "VAR总磷总氮全局变量.vi" "MB session in"() -> (w159:refnum<class "MB_Master.lvclass">)
        n141 = call "版本判断.vi"() -> ("仪器版本"=w160:T9)  [unwired: 11 in]
        n142 = case shown="\"V4.2版\"" w160 {
          tunnel: w159 -> [w168 w175 w182 w189]
          tunnel: w158 -> [w163 w171 w178 w185]
          tunnel: [w162 w169 w176 w183] -> w157
          frame "V3.1版", Default {
            n143 = call "读取V3.1外设配置.vi"("MB session in"=w168) -> ("error out"=w164:errorcluster, "外设配置"=w167:T10, "MB session out"=w166:refnum<class "MB_Master.lvclass">)  [unwired: 8 in]
            n144 = Bundle By Name(cluster=w167, "消解温度下限"=w163) -> (w165:T10)
            n145 = call "写入V3.1外设配置.vi"("error in (no error)"=w164, "外设配置"=w165, "MB session in"=w166) -> ("error out"=w162:errorcluster)  [unwired: 7 in, 1 out]
          }
          frame "V4版" {
            n146 = call "读取V4版外设配置.vi"("MB session in"=w175) -> ("error out"=w170:errorcluster, "外设配置"=w173:T11, "MB session out"=w174:refnum<class "MB_Master.lvclass">)  [unwired: 8 in]
            n147 = Bundle By Name(cluster=w173, "消解温度下限"=w171) -> (w172:T11)
            n148 = call "写入V4版外设配置.vi"("error in (no error)"=w170, "外设配置"=w172, "MB session in"=w174) -> ("error out"=w169:errorcluster)  [unwired: 7 in, 1 out]
          }
          frame "V4.2版" {
            n149 = call "读取V4.2版外设配置.vi"("MB session in"=w182) -> ("error out"=w177:errorcluster, "外设配置"=w180:T12, "MB session out"=w181:refnum<class "MB_Master.lvclass">)  [unwired: 8 in]
            n150 = Bundle By Name(cluster=w180, "消解温度"=w178) -> (w179:T12)
            n151 = call "写入V4.2版外设配置.vi"("error in (no error)"=w177, "外设配置"=w179, "MB session in"=w181) -> ("error out"=w176:errorcluster)  [unwired: 7 in, 1 out]
          }
          frame "V3版" {
            n152 = call "读取V3外设配置.vi"("MB session in"=w189) -> ("error out"=w184:errorcluster, "外设配置"=w187:T13, "MB session out"=w188:refnum<class "MB_Master.lvclass">)  [unwired: 8 in]
            n153 = Bundle By Name(cluster=w187, "消解温度下限"=w185) -> (w186:T13)
            n154 = call "写入V3外设配置.vi"("error in (no error)"=w184, "外设配置"=w186, "MB session in"=w188) -> ("error out"=w183:errorcluster)  [unwired: 7 in, 1 out]
          }
        }
        n155 = case shown="Error" w157 {
          tunnel: ["写入成功" "写入失败"] -> w161
          frame No Error {
          }
          frame Error {
          }
        }
        n156 = One Button Dialog(message=w161) -> ()  [unwired: 1 in, 1 out]
      }
      event "测量精度": Mouse Down {
        n157 = event-data() -> ("CtlRef"=w193:refnum<vi>)  [unwired: 1 in, 7 out]
        n158 = global read "VAR总磷总氮全局变量.vi" "权限等级"() -> (w192:enum16{"一级权限", "二级权限", "三级权限", "超级权限"})
        n159 = case shown="\"二级权限\"..\"超级权限\"" w192 {
          tunnel: w193 -> [_ w197]
          frame "一级权限", Default {
          }
          frame "二级权限".."超级权限" {
            n160 = property class="DigNum (strict)"(reference=w197) -> (reference out=w195:refnum<vi>, "Value"=w196:u16)  [unwired: 1 in, 1 out]
            n161 = call "数字键盘.vi"("OldNumber"=w196) -> ("NewNumber"=w194:dbl)
            n162 = property class="DigNum (strict)"(reference=w195, "Val(Sgnl)"=w194) -> ()  [unwired: 1 in, 2 out]
          }
        }
      }
      event "盐度补偿值": Mouse Down {
        n163 = event-data() -> ("CtlRef"=w199:refnum<vi>)  [unwired: 1 in, 3 out]
        n164 = global read "VAR总磷总氮全局变量.vi" "权限等级"() -> (w198:enum16{"一级权限", "二级权限", "三级权限", "超级权限"})
        n165 = case shown="\"二级权限\"..\"超级权限\"" w198 {
          tunnel: w199 -> [_ w201]
          frame "一级权限", Default {
          }
          frame "二级权限".."超级权限" {
            n166 = case shown="False" "盐度自动补偿：" {
              tunnel: w201 -> [w205 _]
              frame False {
                n167 = property class="DigNum (strict)"(reference=w205) -> (reference out=w203:refnum<vi>, "Value"=w204:dbl)  [unwired: 1 in, 1 out]
                n168 = call "数字键盘.vi"("OldNumber"=w204) -> ("NewNumber"=w202:dbl)
                n169 = property class="DigNum (strict)"(reference=w203, "Val(Sgnl)"=w202) -> ()  [unwired: 1 in, 2 out]
              }
              frame True {
              }
            }
          }
        }
      }
      event "盐度补偿值": Value Change {
        n170 = event-data() -> ("NewVal"=w206:dbl)  [unwired: 1 in, 5 out]
        n171 = global read "VAR总磷总氮全局变量.vi" "MB session in"() -> (w207:refnum<class "MB_Master.lvclass">)
        n172 = call "盐度补偿值写入.vi"("盐度补偿值"=w206, "MB session in"=w207) -> ()  [unwired: 8 in, 2 out]
      }
      event "跨度值", "零点核查标液浓度", "跨度核查标液浓度", "标样核查标液浓度", "消解时长", "测试流程路径", "盐度自动补偿：", "IP", "PORT", "请选择串口:", "通信方式选择", "简易流程路径", "低量程上限", "零点核查标液偏差", "跨度核查标液偏差", "标样核查标液偏差", "零点核查自动补测", "跨度核查自动补测", "标样核查自动补测", "协议", "波   特   率:": Value Change {
        n173 = event-data() -> ()  [unwired: 1 in, 6 out]
        n174 = global read "VAR总磷总氮全局变量.vi" "权限等级"() -> (w209:enum16{"一级权限", "二级权限", "三级权限", "超级权限"})
        n175 = case shown="\"二级权限\"..\"超级权限\"" w209 {
          tunnel: w210 -> [_ w212]
          tunnel: w208 -> [w211 _]
          frame "一级权限", Default {
            n176 = Set Occurrence(w211) -> ()
          }
          frame "二级权限".."超级权限" {
            n177 = flat-sequence {
              tunnel: w212 -> [w244]
              frame #0 {
                n178 = property class="Ring (strict)"(reference=w244) -> ("Value"=w243:u16)  [unwired: 1 in, 2 out]
                n179 = local read "通信方式选择"() -> (w226:enum16{"串口", "TCP"})
                n180 = local read "盐度自动补偿："() -> (w230:bool)
                n181 = global write "总磷总氮断电保存全局变量.vi" "MB通信方式选择"(w226) -> ()
                n182 = Bundle("水样测试量程模式"="水样测试量程模式", "零点核查量程模式"="零点核查量程模式", "跨度核查量程模式"="跨度核查量程模式", "加标回收量程模式"="加标回收量程模式", "标样核查量程模式"="标样核查量程模式") -> (w232:T14)  [unwired: 1 in]
                n183 = global write "总磷总氮断电保存全局变量.vi" "简易流程路径"("简易流程路径") -> ()
                n184 = global write "总磷总氮断电保存全局变量.vi" "IP"("IP") -> ()
                n185 = global write "总磷总氮断电保存全局变量.vi" "盐度自动补偿："(w230) -> ()
                n186 = global write "总磷总氮断电保存全局变量.vi" "流程路径"("测试流程路径") -> ()
                n187 = global write "总磷总氮断电保存全局变量.vi" "标样核查自动补测"("标样核查自动补测") -> ()
                n188 = global write "总磷总氮断电保存全局变量.vi" "PORT"("PORT") -> ()
                n189 = global write "总磷总氮断电保存全局变量.vi" "跨度核查自动补测"("跨度核查自动补测") -> ()
                n190 = global write "总磷总氮断电保存全局变量.vi" "VISA Resource"("请选择串口:") -> ()
                n191 = global write "总磷总氮断电保存全局变量.vi" "零点核查自动补测"("零点核查自动补测") -> ()
                n192 = global write "总磷总氮断电保存全局变量.vi" "波特率"("波   特   率:") -> ()
                n193 = global write "总磷总氮断电保存全局变量.vi" "协议"("协议") -> ()
                n194 = To Unsigned Word Integer(number=w232) -> (unsigned 16bit integer=w231:cluster{u16, u16, u16, u16, u16})
                n195 = global read "总磷总氮断电保存全局变量.vi" "低量程上限"() -> (w223:T15)
                n196 = property on="低量程上限" class="DigNum (strict)"() -> ("Value"=w221:dbl)  [unwired: 2 in, 2 out]
                n197 = global read "总磷总氮断电保存全局变量.vi" "质控参数设置"() -> (w238:T16)
                n198 = local read "消解时长"() -> (w225:dbl)
                n199 = case shown="1" w243 {
                  tunnel: "跨度值" -> [_ w258 w272 w285 w298 w311 w324 w337 w350 w364 w378 w391]
                  tunnel: "标样核查标液浓度" -> [_ w255 w269 w282 w295 w308 w321 w334 w347 w361 w375 w388]
                  tunnel: "跨度核查标液浓度" -> [_ w256 w270 w283 w296 w309 w322 w335 w348 w362 w376 w389]
                  tunnel: "零点核查标液浓度" -> [_ w257 w271 w284 w297 w310 w323 w336 w349 w363 w377 w390]
                  tunnel: w238 -> [_ w260 w274 w287 w300 w313 w326 w339 w352 w366 w380 w393]
                  tunnel: w231 -> [_ w254 w268 w281 w294 w307 w320 w333 w346 w359 w373 w387]
                  tunnel: w225 -> [_ w253 w267 _ _ _ _ _ _ w360 w374 _]
                  tunnel: w223 -> [w246 w251 w266 w280 w293 w306 w319 w332 w345 w358 w372 w386]
                  tunnel: [w246 w250 w264 w279 w292 w305 w318 w331 w344 w357 w371 w385] -> w222
                  tunnel: w221 -> [_ w252 w265 w278 w291 w304 w317 w330 w343 w356 w370 w384]
                  tunnel: "标样核查标液偏差" -> [_ w249 w261 w275 w288 w303 w314 w327 w340 w353 w367 w381]
                  tunnel: "跨度核查标液偏差" -> [_ w248 w262 w276 w289 w302 w315 w328 w341 w354 w368 w382]
                  tunnel: "零点核查标液偏差" -> [_ w247 w263 w277 w290 w301 w316 w329 w342 w355 w369 w383]
                  frame 0, Default {
                  }
                  frame 1 {
                    n200 = global write "总磷总氮断电保存全局变量.vi" "总磷自动测试量程配置"(w254) -> ()
                    n201 = global write "总磷总氮断电保存全局变量.vi" "总磷消解时长"(w253) -> ()
                    n202 = Bundle By Name(cluster=w251, "总磷"=w252) -> (w250:T15)
                    n203 = Bundle By Name(cluster=w260, "总磷跨度值"=w258, "总磷零点标准液浓度"=w257, "总磷跨度标准液浓度"=w256, "总磷标准液标准浓度"=w255, "总磷零点标准液偏差"=w247, "总磷跨度标准液偏差"=w248, "总磷标准液标准偏差"=w249) -> (w259:T16)
                    n204 = global write "总磷总氮断电保存全局变量.vi" "质控参数设置"(w259) -> ()
                  }
                  frame 2 {
                    n205 = global write "总磷总氮断电保存全局变量.vi" "总氮自动测试量程配置"(w268) -> ()
                    n206 = global write "总磷总氮断电保存全局变量.vi" "总氮消解时长"(w267) -> ()
                    n207 = Bundle By Name(cluster=w266, "总氮"=w265) -> (w264:T15)
                    n208 = Bundle By Name(cluster=w274, "总氮跨度值"=w272, "总氮零点标准液浓度"=w271, "总氮跨度标准液浓度"=w270, "总氮标准液标准浓度"=w269, "总氮零点标准液偏差"=w263, "总氮跨度标准液偏差"=w262, "总氮标准液标准偏差"=w261) -> (w273:T16)
                    n209 = global write "总磷总氮断电保存全局变量.vi" "质控参数设置"(w273) -> ()
                  }
                  frame 3 {
                    n210 = global write "总磷总氮断电保存全局变量.vi" "氨氮自动测试量程配置"(w281) -> ()
                    n211 = Bundle By Name(cluster=w280, "氨氮"=w278) -> (w279:T15)
                    n212 = Bundle By Name(cluster=w287, "氨氮跨度值"=w285, "氨氮零点标准液浓度"=w284, "氨氮跨度标准液浓度"=w283, "氨氮标准液标准浓度"=w282, "氨氮零点标准液偏差"=w277, "氨氮跨度标准液偏差"=w276, "氨氮标准液标准偏差"=w275) -> (w286:T16)
                    n213 = global write "总磷总氮断电保存全局变量.vi" "质控参数设置"(w286) -> ()
                  }
                  frame 4 {
                    n214 = global write "总磷总氮断电保存全局变量.vi" "磷酸盐自动测试量程配置"(w294) -> ()
                    n215 = Bundle By Name(cluster=w293, "磷酸盐"=w291) -> (w292:T15)
                    n216 = Bundle By Name(cluster=w300, "磷酸盐跨度值"=w298, "磷酸盐零点标准液浓度"=w297, "磷酸盐跨度标准液浓度"=w296, "磷酸盐标准液标准浓度"=w295, "磷酸盐零点标准液偏差"=w290, "磷酸盐跨度标准液偏差"=w289, "磷酸盐标准液标准偏差"=w288) -> (w299:T16)
                    n217 = global write "总磷总氮断电保存全局变量.vi" "质控参数设置"(w299) -> ()
                  }
                  frame 5 {
                    n218 = global write "总磷总氮断电保存全局变量.vi" "硝氮自动测试量程配置"(w307) -> ()
                    n219 = Bundle By Name(cluster=w306, "硝氮"=w304) -> (w305:T15)
                    n220 = Bundle By Name(cluster=w313, "硝氮跨度值"=w311, "硝氮零点标准液浓度"=w310, "硝氮跨度标准液浓度"=w309, "硝氮标准液标准浓度"=w308, "硝氮零点标准液偏差"=w301, "硝氮跨度标准液偏差"=w302, "硝氮标准液标准偏差"=w303) -> (w312:T16)
                    n221 = global write "总磷总氮断电保存全局变量.vi" "质控参数设置"(w312) -> ()
                  }
                  frame 6 {
                    n222 = global write "总磷总氮断电保存全局变量.vi" "亚硝氮自动测试量程配置"(w320) -> ()
                    n223 = Bundle By Name(cluster=w319, "亚硝氮"=w317) -> (w318:T15)
                    n224 = Bundle By Name(cluster=w326, "亚硝氮跨度值"=w324, "亚硝氮零点标准液浓度"=w323, "亚硝氮跨度标准液浓度"=w322, "亚硝氮标准液标准浓度"=w321, "亚硝氮零点标准液偏差"=w316, "亚硝氮跨度标准液偏差"=w315, "亚硝氮标准液标准偏差"=w314) -> (w325:T16)
                    n225 = global write "总磷总氮断电保存全局变量.vi" "质控参数设置"(w325) -> ()
                  }
                  frame 7 {
                    n226 = global write "总磷总氮断电保存全局变量.vi" "硅酸盐自动测试量程配置"(w333) -> ()
                    n227 = Bundle By Name(cluster=w332, "硅酸盐"=w330) -> (w331:T15)
                    n228 = Bundle By Name(cluster=w339, "硅酸盐跨度值"=w337, "硅酸盐零点标准液浓度"=w336, "硅酸盐跨度标准液浓度"=w335, "硅酸盐标准液标准浓度"=w334, "硅酸盐零点标准液偏差"=w329, "硅酸盐跨度标准液偏差"=w328, "硅酸盐标准液标准偏差"=w327) -> (w338:T16)
                    n229 = global write "总磷总氮断电保存全局变量.vi" "质控参数设置"(w338) -> ()
                  }
                  frame 8 {
                    n230 = global write "总磷总氮断电保存全局变量.vi" "硫化物自动测试量程配置"(w346) -> ()
                    n231 = Bundle By Name(cluster=w345, "硫化物"=w343) -> (w344:T15)
                    n232 = Bundle By Name(cluster=w352, "硫化物跨度值"=w350, "硫化物零点标准液浓度"=w349, "硫化物跨度标准液浓度"=w348, "硫化物标准液标准浓度"=w347, "硫化物零点标准液偏差"=w342, "硫化物跨度标准液偏差"=w341, "硫化物标准液标准偏差"=w340) -> (w351:T16)
                    n233 = global write "总磷总氮断电保存全局变量.vi" "质控参数设置"(w351) -> ()
                  }
                  frame 22 {
                    n234 = global write "总磷总氮断电保存全局变量.vi" "COD自动测试量程配置"(w359) -> ()
                    n235 = global write "总磷总氮断电保存全局变量.vi" "CODcr消解时长"(w360) -> ()
                    n236 = Bundle By Name(cluster=w358, "COD"=w356) -> (w357:T15)
                    n237 = Bundle By Name(cluster=w366, "COD跨度值"=w364, "COD零点标准液浓度"=w363, "COD跨度标准液浓度"=w362, "COD标准液标准浓度"=w361, "COD零点标准液偏差"=w355, "COD跨度标准液偏差"=w354, "COD标准液标准偏差"=w353) -> (w365:T16)
                    n238 = global write "总磷总氮断电保存全局变量.vi" "质控参数设置"(w365) -> ()
                  }
                  frame 21 {
                    n239 = global write "总磷总氮断电保存全局变量.vi" "CODMn自动测试量程配置"(w373) -> ()
                    n240 = global write "总磷总氮断电保存全局变量.vi" "CODmn消解时长"(w374) -> ()
                    n241 = Bundle By Name(cluster=w372, "CODMn"=w370) -> (w371:T15)
                    n242 = Bundle By Name(cluster=w380, "CODMn跨度值"=w378, "CODMn零点标准液浓度"=w377, "CODMn跨度标准液浓度"=w376, "CODMn标准液标准浓度"=w375, "CODMn零点标准液偏差"=w369, "CODMn跨度标准液偏差"=w368, "CODMn标准液标准偏差"=w367) -> (w379:T16)
                    n243 = global write "总磷总氮断电保存全局变量.vi" "质控参数设置"(w379) -> ()
                  }
                  frame 50 {
                    n244 = global write "总磷总氮断电保存全局变量.vi" "氟化物自动测试量程配置"(w387) -> ()
                    n245 = Bundle By Name(cluster=w386, "氟化物"=w384) -> (w385:T15)
                    n246 = Bundle By Name(cluster=w393, "氟化物跨度值"=w391, "氟化物零点标准液浓度"=w390, "氟化物跨度标准液浓度"=w389, "氟化物标准液标准浓度"=w388, "氟化物零点标准液偏差"=w383, "氟化物跨度标准液偏差"=w382, "氟化物标准液标准偏差"=w381) -> (w392:T16)
                    n247 = global write "总磷总氮断电保存全局变量.vi" "质控参数设置"(w392) -> ()
                  }
                }
                n248 = global write "总磷总氮断电保存全局变量.vi" "低量程上限"(w222) -> ()
              }
              frame #1 {
                n249 = Get Date/Time In Seconds() -> (seconds since 1Jan1904=w396:timestamp)
                n250 = property on="参数下拉列表" class="Ring (strict)"() -> ("RingText.Text"=w394:string)  [unwired: 2 in, 2 out]
                n251 = Bundle By Name(cluster=T8 {"时间"=timestamp(0 s since 1904-01-01), "参数"="", "日志信息"="", "流程参数"=""} ("data in"), "时间"=w396, "参数"=w394, "日志信息"="参数变更") -> (w397:T8)
                n252 = call "总磷总氮操作日志.vi"("data in"=w397) -> ()  [unwired: 10 in, 1 out]
                n253 = call "仪器配置写入.vi"() -> ()  [unwired: 11 in, 1 out]
              }
            }
          }
        }
      }
      event "通讯连接": Value Change {
        n254 = event-data() -> ("NewVal"=w399:bool)  [unwired: 1 in, 5 out]
        n255 = Flush Queue(queue=w400) -> (queue out=w401:refnum<queue>)  [unwired: 1 in, 2 out]
        n256 = case shown="False" w399 {
          tunnel: w401 -> [w402 w404]
          frame False {
            n257 = Enqueue Element At Opposite End(queue=w402, element=cluster{"命令":string, "data":variant} {"命令"="停用模块", "data"=variant} ("元素")) -> ()  [unwired: 2 in, 3 out]
          }
          frame True {
            n258 = Enqueue Element At Opposite End(queue=w404, element=cluster{"命令":string, "data":variant} {"命令"="启用模块", "data"=variant} ("元素")) -> ()  [unwired: 2 in, 3 out]
          }
        }
      }
      event "手动模式": Value Change {
        n259 = event-data() -> ()  [unwired: 1 in, 6 out]
        n260 = global write "VAR总磷总氮全局变量.vi" "手动模式"("手动模式") -> ()
      }
    }
  }
  n261 = while {
    tunnel: w7 -> [w417]
    tunnel: w8 -> [w416]
    tunnel: w9 -> [w415]
    tunnel: w6 -> [w414]
    stop <- FALSE stop-if-true
    n262 = Wait on Occurrence(2:w414) -> (0:w408:bool)  [unwired: 2 in]
    n263 = flat-sequence {
      tunnel: w417 -> [w424]
      tunnel: w416 -> [w423]
      tunnel: w415 -> [w422]
      tunnel: [w421] -> w411
      tunnel: [w420] -> w410
      tunnel: [w419] -> w409
      tunnel: w408 -> [_]
      frame #0 {
        n264 = property class="Enum (strict)"(reference=w423) -> ("Value"=w420:enum16{"低量程", "高量程"})  [unwired: 1 in, 2 out]
        n265 = property class="Ring (strict)"(reference=w424) -> ("Value"=w421:u16)  [unwired: 1 in, 2 out]
        n266 = property class="Enum (strict)"(reference=w422) -> ("Value"=w419:T1)  [unwired: 1 in, 2 out]
      }
    }
    n267 = flat-sequence {
      tunnel: [w427] -> w413
      tunnel: [w426] -> w412
      tunnel: w411 -> [w425]
      tunnel: w410 -> [w427]
      tunnel: w409 -> [w426]
      tunnel: [w425] -> w407
      tunnel: w413 -> [w442]
      tunnel: w412 -> [w443]
      tunnel: w407 -> [w441]
      frame #0 {
      }
      frame #1 {
        n268 = global read "总磷总氮断电保存全局变量.vi" "协议"() -> (w428:u16)
        n269 = case shown="2, Default" w428 {
          tunnel: w443 -> [_ w496]
          tunnel: w442 -> [_ w495]
          tunnel: w441 -> [_ w494]
          tunnel: [w455 w492] -> w440
          tunnel: [w454 w491] -> w439
          tunnel: [_ w490] -> w438
          tunnel: [w451 w489] -> w437
          tunnel: [_ w488] -> w436
          tunnel: [_ w487] -> w435
          tunnel: [_ w486] -> w434
          tunnel: [w450 w483] -> w433
          tunnel: [w449 w482] -> w432
          tunnel: [w448 w481] -> w431
          tunnel: [w447 w480] -> w430
          tunnel: [w446 w477] -> w429
          frame 2, Default {
            n270 = global read "VAR总磷总氮全局变量.vi" "MB session in"() -> (w456:refnum<class "MB_Master.lvclass">)
            n271 = call <vilib>:"Read Holding Registers.vi"("quantity"=u16 56, "starting address"=u16 4256, "MB session in"=w456) -> ("error out"=w466:errorcluster, "Registers"=w445:u16[], "MB session out"=w472:refnum<class "MB_Master.lvclass">)  [unwired: 6 in]
            n272 = call "关键参数区.vi"("数组"=w445) -> ("关键参数区"=w444:T17)  [unwired: 10 in]
            n273 = call <vilib>:"Read Holding Registers.vi"("error in (no error)"=w466, "quantity"=u16 2, "starting address"=u16 256, "MB session in"=w472) -> ("error out"=w457:errorcluster, "Registers"=w469:u16[], "MB session out"=w465:refnum<class "MB_Master.lvclass">)  [unwired: 5 in]
            n274 = Unbundle By Name(w444) -> ("测量精度"=w455:u16, "检出限值"=w454:sgl, "消解时长"=w453:u16, "量程下限"=w451:sgl, "量程上限"=w452:sgl, "曲线斜率K"=w449:sgl, "曲线斜率B"=w448:sgl, "消解温度"=w447:u16)
            n275 = call <vilib>:"Read Holding Registers.vi"("error in (no error)"=w457, "quantity"=u16 2, "starting address"=u16 4312, "MB session in"=w465) -> ("Registers"=w458:u16[])  [unwired: 5 in, 2 out]
            n276 = Type Cast(type=u32 0, x=w469) -> (*(type *) &x=w471:u32)
            n277 = Swap Words(1:w471) -> (0:w470:u32)
            n278 = Type Cast(type=u32 0, x=w458) -> (*(type *) &x=w459:u32)
            n279 = Swap Words(1:w459) -> (0:w460:u32)
            n280 = local write "消解时长"(w453) -> ()
            n281 = local write "低量程上限"(w452) -> ()
            n282 = Type Cast(type=sgl 0.0, x=w470) -> (*(type *) &x=w446:sgl)
            n283 = Type Cast(type=sgl 0.0, x=w460) -> (*(type *) &x=w450:sgl)
          }
          frame 1 {
            n284 = call "量程参数读取.vi"("测量参数"=w494) -> ("error out"=w485:errorcluster, "量程参数读取"=w493:T7)  [unwired: 9 in]
            n285 = Unbundle By Name(w493) -> ("测量精度"=w492:u16, "检出限"=w491:dbl, "上限"=w490:dbl, "下限"=w489:dbl, "阈值（低->高）"=w488:dbl, "阈值（高->低）"=w487:dbl, "稀释度"=w486:dbl)
            n286 = call "公式读取.vi"("error in (no error)"=w485, "量程"=w495, "测量模式"=w496, "测量参数"=w494) -> ("error out"=w479:errorcluster, "公式"=w484:cluster{"X^2":dbl, "X":dbl, "b":dbl})  [unwired: 6 in]
            n287 = Unbundle By Name(w484) -> ("X^2"=w483:dbl, "X"=w482:dbl, "b"=w481:dbl)
            n288 = global read "VAR总磷总氮全局变量.vi" "MB session in"() -> (w478:refnum<class "MB_Master.lvclass">)
            n289 = case shown="1, 2, 21, 22" w494 {
              tunnel: [_ w499] -> w480
              tunnel: [w497 w505] -> _
              tunnel: w479 -> [w497 w500]
              tunnel: w478 -> [_ w503]
              tunnel: [_ w504] -> w477
              frame 0, Default {
              }
              frame 1, 2, 21, 22 {
                n290 = call "版本判断.vi"() -> ("仪器版本"=w502:T9)  [unwired: 11 in]
                n291 = case shown="\"V4.2版\"" w502 {
                  tunnel: [w511 w515 w520 w526] -> w501
                  tunnel: w503 -> [w510 w516 w521 w527]
                  tunnel: [w507 w513 w518 w524] -> w499
                  tunnel: w500 -> [w509 _ _ w523]
                  tunnel: [w506 w512 w517 w522] -> w498
                  frame "V3.1版", Default {
                    n292 = call "读取V3.1外设配置.vi"("error in (no error)"=w509, "MB session in"=w510) -> ("error out"=w511:errorcluster, "外设配置"=w508:T10, "MB session out"=w506:refnum<class "MB_Master.lvclass">)  [unwired: 7 in]
                    n293 = Unbundle By Name(w508) -> ("消解温度下限"=w507:sgl)
                  }
                  frame "V4版" {
                    n294 = call "读取V4版外设配置.vi"("MB session in"=w516) -> ("error out"=w515:errorcluster, "外设配置"=w514:T11, "MB session out"=w512:refnum<class "MB_Master.lvclass">)  [unwired: 8 in]
                    n295 = Unbundle By Name(w514) -> ("消解温度下限"=w513:sgl)
                  }
                  frame "V4.2版" {
                    n296 = call "读取V4.2版外设配置.vi"("MB session in"=w521) -> ("error out"=w520:errorcluster, "外设配置"=w519:T12, "MB session out"=w517:refnum<class "MB_Master.lvclass">)  [unwired: 8 in]
                    n297 = Unbundle By Name(w519) -> ("消解温度"=w518:sgl)
                  }
                  frame "V3版" {
                    n298 = call "读取V3外设配置.vi"("error in (no error)"=w523, "MB session in"=w527) -> ("error out"=w526:errorcluster, "外设配置"=w525:T13, "MB session out"=w522:refnum<class "MB_Master.lvclass">)  [unwired: 7 in]
                    n299 = Unbundle By Name(w525) -> ("消解温度下限"=w524:sgl)
                  }
                }
                n300 = call "盐度补偿值读取.vi"("Error in"=w501, "MB session in"=w498) -> ("error out"=w505:errorcluster, "盐度补偿值"=w504:sgl)  [unwired: 7 in, 1 out]
              }
            }
          }
        }
        "测量精度" <- w440
        "检出限" <- w439
        "高量程上限" <- w438
        "量程下限" <- w437
        "阈值（低->高）" <- w436
        "阈值（高->低）" <- w435
        "稀释度" <- w434
        "二次多项式系数" <- w433
        "曲线斜率" <- w432
        "曲线截距" <- w431
        "消解温度" <- w430
        "盐度补偿值" <- w429
      }
      frame #2 {
        n301 = Format Date/Time String() -> (date/time string=→"数据刷新时间":string)  [unwired: 3 in]
      }
    }
  }
  n302 = while {
    tunnel: w7 -> [w540]
    stop <- FALSE stop-if-true
    n303 = property class="Ring (strict)"(reference=w540) -> ("Value"=w539:u16)  [unwired: 1 in, 2 out]
    n304 = global read "总磷总氮断电保存全局变量.vi" "盐度自动补偿："() -> (w555:bool)
    n305 = global read "总磷总氮断电保存全局变量.vi" "跨度核查自动补测"() -> (w530:bool)
    n306 = global read "总磷总氮断电保存全局变量.vi" "MB通信方式选择"() -> (w554:enum16{"串口", "TCP"})
    n307 = global read "总磷总氮断电保存全局变量.vi" "VISA Resource"() -> (w559:refnum<visa-resource-name>)
    n308 = global read "总磷总氮断电保存全局变量.vi" "简易流程路径"() -> (w538:path)
    n309 = global read "总磷总氮断电保存全局变量.vi" "零点核查自动补测"() -> (w532:bool)
    n310 = global read "总磷总氮断电保存全局变量.vi" "标样核查自动补测"() -> (w531:bool)
    n311 = global read "总磷总氮断电保存全局变量.vi" "流程路径"() -> (w556:path)
    n312 = global read "总磷总氮断电保存全局变量.vi" "PORT"() -> (w558:string)
    n313 = local write "盐度自动补偿："(w555) -> ()
    n314 = global read "总磷总氮断电保存全局变量.vi" "质控参数设置"() -> (w549:T16)
    n315 = global read "总磷总氮断电保存全局变量.vi" "低量程上限"() -> (w537:T15)
    n316 = local write "跨度核查自动补测"(w530) -> ()
    n317 = local write "通信方式选择"(w554) -> ()
    n318 = local write "请选择串口:"(w559) -> ()
    n319 = local write "简易流程路径"(w538) -> ()
    n320 = local write "零点核查自动补测"(w532) -> ()
    n321 = local write "标样核查自动补测"(w531) -> ()
    n322 = local write "测试流程路径"(w556) -> ()
    n323 = local write "PORT"(w558) -> ()
    n324 = case shown="21" w539 {
      tunnel: [_ w576 w588 w599 w610 w621 w632 w643 w654 w666 w677 w689] -> w547
      tunnel: [_ w575 w587 _ _ _ _ _ _ w665 _ w678] -> w548
      tunnel: w549 -> [_ w574 w586 w598 w609 w620 w631 w642 w653 w664 w676 w688]
      tunnel: [_ w573 w585 w597 w608 w619 w630 w641 w652 w663 w675 w687] -> w550
      tunnel: [_ w572 w584 w596 w607 w618 w629 w640 w651 w662 w674 w686] -> w551
      tunnel: [_ w571 w583 w595 w606 w617 w628 w639 w650 w661 w673 w685] -> w552
      tunnel: [_ w570 w582 w594 w605 w616 w627 w638 w649 w660 w672 w684] -> w553
      tunnel: w537 -> [_ w569 w581 w593 w604 w615 w626 w637 w648 w659 w671 w683]
      tunnel: [0.0 ("COD") w568 w580 w592 w603 w614 w625 w636 w647 w658 w670 w682] -> w536
      tunnel: [_ w567 w579 w591 w602 w613 w624 w635 w646 w657 w669 w681] -> w535
      tunnel: [_ w566 w578 w590 w601 w612 w623 w634 w645 w656 w668 w680] -> w534
      tunnel: [_ w565 w577 w589 w600 w611 w622 w633 w644 w655 w667 w679] -> w533
      frame Default {
      }
      frame 1 {
        n325 = Unbundle By Name(w574) -> ("总磷跨度值"=w573:dbl, "总磷零点标准液浓度"=w572:dbl, "总磷跨度标准液浓度"=w571:dbl, "总磷标准液标准浓度"=w570:dbl, "总磷零点标准液偏差"=w567:dbl, "总磷跨度标准液偏差"=w566:dbl, "总磷标准液标准偏差"=w565:dbl)
        n326 = Unbundle By Name(w569) -> ("总磷"=w568:dbl)
        n327 = global read "总磷总氮断电保存全局变量.vi" "总磷消解时长"() -> (w575:dbl)
        n328 = global read "总磷总氮断电保存全局变量.vi" "总磷自动测试量程配置"() -> (w576:T18)
      }
      frame 2 {
        n329 = Unbundle By Name(w586) -> ("总氮跨度值"=w585:dbl, "总氮零点标准液浓度"=w584:dbl, "总氮跨度标准液浓度"=w583:dbl, "总氮标准液标准浓度"=w582:dbl, "总氮零点标准液偏差"=w579:dbl, "总氮跨度标准液偏差"=w578:dbl, "总氮标准液标准偏差"=w577:dbl)
        n330 = Unbundle By Name(w581) -> ("总氮"=w580:dbl)
        n331 = global read "总磷总氮断电保存全局变量.vi" "总氮消解时长"() -> (w587:dbl)
        n332 = global read "总磷总氮断电保存全局变量.vi" "总氮自动测试量程配置"() -> (w588:T18)
      }
      frame 3 {
        n333 = Unbundle By Name(w598) -> ("氨氮跨度值"=w597:dbl, "氨氮零点标准液浓度"=w596:dbl, "氨氮跨度标准液浓度"=w595:dbl, "氨氮标准液标准浓度"=w594:dbl, "氨氮零点标准液偏差"=w591:dbl, "氨氮跨度标准液偏差"=w590:dbl, "氨氮标准液标准偏差"=w589:dbl)
        n334 = Unbundle By Name(w593) -> ("氨氮"=w592:dbl)
        n335 = global read "总磷总氮断电保存全局变量.vi" "氨氮自动测试量程配置"() -> (w599:T18)
      }
      frame 4 {
        n336 = Unbundle By Name(w609) -> ("磷酸盐跨度值"=w608:dbl, "磷酸盐零点标准液浓度"=w607:dbl, "磷酸盐跨度标准液浓度"=w606:dbl, "磷酸盐标准液标准浓度"=w605:dbl, "磷酸盐零点标准液偏差"=w602:dbl, "磷酸盐跨度标准液偏差"=w601:dbl, "磷酸盐标准液标准偏差"=w600:dbl)
        n337 = Unbundle By Name(w604) -> ("磷酸盐"=w603:dbl)
        n338 = global read "总磷总氮断电保存全局变量.vi" "磷酸盐自动测试量程配置"() -> (w610:T18)
      }
      frame 5 {
        n339 = Unbundle By Name(w620) -> ("硝氮跨度值"=w619:dbl, "硝氮零点标准液浓度"=w618:dbl, "硝氮跨度标准液浓度"=w617:dbl, "硝氮标准液标准浓度"=w616:dbl, "硝氮零点标准液偏差"=w613:dbl, "硝氮跨度标准液偏差"=w612:dbl, "硝氮标准液标准偏差"=w611:dbl)
        n340 = Unbundle By Name(w615) -> ("硝氮"=w614:dbl)
        n341 = global read "总磷总氮断电保存全局变量.vi" "硝氮自动测试量程配置"() -> (w621:T18)
      }
      frame 6 {
        n342 = Unbundle By Name(w631) -> ("亚硝氮跨度值"=w630:dbl, "亚硝氮零点标准液浓度"=w629:dbl, "亚硝氮跨度标准液浓度"=w628:dbl, "亚硝氮标准液标准浓度"=w627:dbl, "亚硝氮零点标准液偏差"=w624:dbl, "亚硝氮跨度标准液偏差"=w623:dbl, "亚硝氮标准液标准偏差"=w622:dbl)
        n343 = Unbundle By Name(w626) -> ("亚硝氮"=w625:dbl)
        n344 = global read "总磷总氮断电保存全局变量.vi" "亚硝氮自动测试量程配置"() -> (w632:T18)
      }
      frame 7 {
        n345 = Unbundle By Name(w642) -> ("硅酸盐跨度值"=w641:dbl, "硅酸盐零点标准液浓度"=w640:dbl, "硅酸盐跨度标准液浓度"=w639:dbl, "硅酸盐标准液标准浓度"=w638:dbl, "硅酸盐零点标准液偏差"=w635:dbl, "硅酸盐跨度标准液偏差"=w634:dbl, "硅酸盐标准液标准偏差"=w633:dbl)
        n346 = Unbundle By Name(w637) -> ("硅酸盐"=w636:dbl)
        n347 = global read "总磷总氮断电保存全局变量.vi" "硅酸盐自动测试量程配置"() -> (w643:T18)
      }
      frame 8 {
        n348 = Unbundle By Name(w653) -> ("硫化物跨度值"=w652:dbl, "硫化物零点标准液浓度"=w651:dbl, "硫化物跨度标准液浓度"=w650:dbl, "硫化物标准液标准浓度"=w649:dbl, "硫化物零点标准液偏差"=w646:dbl, "硫化物跨度标准液偏差"=w645:dbl, "硫化物标准液标准偏差"=w644:dbl)
        n349 = Unbundle By Name(w648) -> ("硫化物"=w647:dbl)
        n350 = global read "总磷总氮断电保存全局变量.vi" "硫化物自动测试量程配置"() -> (w654:T18)
      }
      frame 22 {
        n351 = Unbundle By Name(w664) -> ("COD跨度值"=w663:dbl, "COD零点标准液浓度"=w662:dbl, "COD跨度标准液浓度"=w661:dbl, "COD标准液标准浓度"=w660:dbl, "COD零点标准液偏差"=w657:dbl, "COD跨度标准液偏差"=w656:dbl, "COD标准液标准偏差"=w655:dbl)
        n352 = Unbundle By Name(w659) -> ("COD"=w658:dbl)
        n353 = global read "总磷总氮断电保存全局变量.vi" "CODcr消解时长"() -> (w665:dbl)
        n354 = global read "总磷总氮断电保存全局变量.vi" "COD自动测试量程配置"() -> (w666:T18)
      }
      frame 50 {
        n355 = Unbundle By Name(w676) -> ("氟化物跨度值"=w675:dbl, "氟化物零点标准液浓度"=w674:dbl, "氟化物跨度标准液浓度"=w673:dbl, "氟化物标准液标准浓度"=w672:dbl, "氟化物零点标准液偏差"=w669:dbl, "氟化物跨度标准液偏差"=w668:dbl, "氟化物标准液标准偏差"=w667:dbl)
        n356 = Unbundle By Name(w671) -> ("氟化物"=w670:dbl)
        n357 = global read "总磷总氮断电保存全局变量.vi" "氟化物自动测试量程配置"() -> (w677:T18)
      }
      frame 21 {
        n358 = Unbundle By Name(w688) -> ("CODMn跨度值"=w687:dbl, "CODMn零点标准液浓度"=w686:dbl, "CODMn跨度标准液浓度"=w685:dbl, "CODMn标准液标准浓度"=w684:dbl, "CODMn零点标准液偏差"=w681:dbl, "CODMn跨度标准液偏差"=w680:dbl, "CODMn标准液标准偏差"=w679:dbl)
        n359 = Unbundle By Name(w683) -> ("CODMn"=w682:dbl)
        n360 = global read "总磷总氮断电保存全局变量.vi" "CODMn自动测试量程配置"() -> (w689:T18)
        n361 = global read "总磷总氮断电保存全局变量.vi" "CODcr消解时长"() -> (w678:dbl)
      }
    }
    n362 = global read "总磷总氮断电保存全局变量.vi" "IP"() -> (w557:string)
    n363 = local write "IP"(w557) -> ()
    n364 = Wait (ms)(milliseconds to wait=u32 1000 ("等待时间（毫秒）")) -> ()  [unwired: 1 out]
    n365 = local write "跨度值"(w550) -> ()
    n366 = local write "零点核查标液浓度"(w551) -> ()
    n367 = local write "跨度核查标液浓度"(w552) -> ()
    n368 = local write "标样核查标液浓度"(w553) -> ()
    n369 = local write "零点核查标液偏差"(w535) -> ()
    n370 = local write "跨度核查标液偏差"(w534) -> ()
    n371 = local write "标样核查标液偏差"(w533) -> ()
    n372 = To Unsigned Word Integer(number=w547) -> (unsigned 16bit integer=w546:T19)
    n373 = global read "总磷总氮断电保存全局变量.vi" "协议"() -> (w529:u16)
    n374 = Unbundle By Name(w546) -> ("水样测试量程模式"=w545:u16, "空白核查量程模式"=w543:u16, "跨度核查量程模式"=w542:u16, "加标回收量程模式"=w541:u16, "标样核查量程模式"=w544:u16)
    n375 = case shown="0, Default" w529 {
      tunnel: w548 -> [_ w563]
      tunnel: w536 -> [_ w562]
      frame 0, Default {
      }
      frame 1 {
        "消解时长" <- w563
        "低量程上限" <- w562
      }
    }
    n376 = local write "水样测试量程模式"(w545) -> ()
    n377 = local write "零点核查量程模式"(w543) -> ()
    n378 = local write "跨度核查量程模式"(w542) -> ()
    n379 = local write "加标回收量程模式"(w541) -> ()
    n380 = local write "标样核查量程模式"(w544) -> ()
  }
